vi "Get All Data Names - When File Is Missing - Returns Error.vi"() -> ()   [LabVIEW 2017, in "Json Data Reader.Tests.lvlib"]
uses:
  Json Data Reader.Tests.lvlib
  Json Data Reader/Json Data Reader.lvclass
  Assertion/Assertion.lvlib
panel:
  out "error out":errorcluster
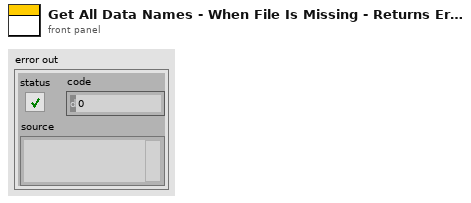
[diagram p1: front panel]
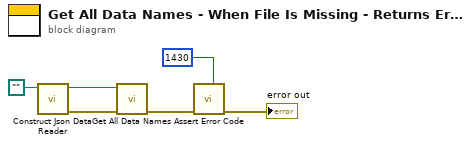
[diagram p0: block diagram]
diagram:
  n1 = call "Construct Json Data Reader.vi"("Json File"=path "") -> ("error out"=w5:errorcluster, "Json Data Reader"=w6:refnum<class "Json Data Reader.lvclass">)  [unwired: 9 in]
  n2 = call "Get All Data Names.vi"("error in (no error)"=w5, "Json Data Reader in"=w6) -> ("error out"=w3:errorcluster)  [unwired: 7 in, 2 out]
  n3 = call "Assert Error Code.vi"("Expected"=1430, "error in (no error)"=w3) -> ("error out"=→"error out":errorcluster)  [unwired: 9 in]
